vi "PopUpDisplay.vi"(0 "Data":i16[][](array[numeric]), 5 "Plane":i32, 7 "Motion Settings In":T1={"No Motion?"=FALSE, "Motion System"=enum."NI 735x", "Motion Bd ID"=1, "Motion Profile"="SMAC1", "# Axis"=1, "Reverse Z axis?"=TRUE, "SMAC Axis"=0, "scan pair"=enum."y-(x) scan", "RT fps"=6.0, "Steps per mm"=[1000, 1000, 1000, 1000], "Motor Parameters"={"velocity ct/s"=[10000.0, 10000.0, 10000.0, 50000.0], "accel ct/s^2"=[50000.0, 50000.0, 50000.0, 200000.0]}, "One Way Scan"=FALSE, "Reverse One Way Scan"=FALSE, "Global Position (mm)"=[], "Plane"=0, "Distance between\nscan lines (um)"=0.0, "Distance between\nscan planes (um)"=0.0, "number of scan planes"=1, "Total steps in line"=0, "Xtra plane\ndistance  (um)"=100, "Xtra planes "=1, "Add Axis"=FALSE, "overshoot cts"=200, "BKPT Shift"=0, "Scan Start Time (ms)"=0, "ESP VISA"="GPIB::1::INSTR", "3rd Axis"=1, "GL Ref Out"=refnum, "Galil Address"=""} {"3rd Axis" items=["x", "y", "z", "w"]; "Xtra planes" min=1; "Xtra plane\ndistance  (um)" min=0; "Distance between\nscan planes (um)" format="%.2f"; "Distance between\nscan lines (um)" format="%.2f"; "SMAC Axis" items=["None"=0, "Axis 1"=1, "Axis 2"=2, "Axis 3"=3, "Axis 4"=4, "Axis 5"=5, "Axis 6"=6, "Axis 7"=7, "Axis 8"=8, "Vector Space 1"=17, "Vector Space 2"=18, "Vector Space 3"=19, "Vector Space 4"=20]; "Motion Bd ID" min=1 max=32 step=1}, 9 "Digitizer Settings":T5={"Digitizer delay (us) "=0.0, "rf points per line"=2048, "lines per plane"=128, "Samp Rate (Hz)"=100000000.0, "Additional dig delay (us)"=0.0, "Voltage Scale"=0.4, "Pre-Looks"=0, "Offset delay (us)"=0.0, "bits A/D"=8, "Avg Num"=1, "DigTimeOut"=5.0, "Rel Dig Delay"=0.0, "Dig Ch"=0, "LeCroyCluster"={"LeCroy Channels"=[TRUE, FALSE, FALSE, FALSE], "LC read pt offset"=0.0, "Sweep Avg"=FALSE}, "Main Digitizer"=enum."NI Digitizer", "Dig Config"=enum."Single channel", "Digitizer ID Cluster"={"Acqiris/Alazar/SP ID"=[], "NI Instr Handles"=[], "LeCroy VISA"="", "GaGe Handle"={"Handle"=0, "Sample size"=0, "Resolution"=0, "Offset"=0, "Channels"=0, "Boards"=0}, "ATS Ref"="ATS9350", "Acqiris Address"=["PCI::INSTR0"], "ADQRef"=refnum, "adq_cu_ptr"=refnum}, "Trigger Settings"={"Trig Source"=1, "Trig Coupling"=0, "Trig Slope"=0, "Level (mV)"=1500.0}, "Bulk Acq"=FALSE, "Bulk Start Indexes"=[], "Data Ref RF"=refnum, "NI ID/Channel"=[], "Total Dig CH"=1, "Xtra Ann Trig delay (us)"=10.0, "Fix Z Delay?"=FALSE, "One Way Transmission?"=FALSE, "Data Ref Log"=refnum} {"Trigger Settings"."Trig Slope" items=["Positive", "Negative"]; "Trigger Settings"."Level (mV)" format="%.2f"; "Trigger Settings"."Trig Coupling" items=["DC 1 MOhm", "AC 1 MOhm", "DC 50 Ohm", "AC 50 Ohm"]; "Trigger Settings"."Trig Source" items=["Chan 1", "External"]; "Rel Dig Delay" format="%.2f"; "DigTimeOut" format="%.2f"; "Avg Num" min=1; "Offset delay (us)" format="%.2f"; "Additional dig delay (us)" format="%.2f"; "Digitizer delay (us)" format="%.2f"}, 11 "virtual T/R Pairs":i32=1) -> ()   [LabVIEW 2022 SP3]
uses:
  ViewData/-ReadEye/ScaleMethod.ctl
  ViewData/-ReadEye/TypeDefs/TypeofMean.ctl
  Digitizers/-DigitizerRoutines/DigitizerSettings.ctl
  Digitizers/-DigitizerRoutines/Digitizer.ctl
  Digitizers/-DigitizerRoutines/DigConfig.ctl
  Digitizers/-DigitizerRoutines/DigitizerID.ctl
  C:/Windows/System32/ADQAPI_dotNet_helper.dll
  Motion Controllers/NI_controller/-NI_MotionRoutines/MotionParameters.ctl
  Motion Controllers/NI_controller/-NI_MotionRoutines/MotionSys.ctl
  Motion Controllers/-MotionRoutines/ScanAxis.ctl
  Motion Controllers/-MotionRoutines/3rdAxis.ctl
  <vilib>/Utility/miscctls.llb/LVRectTypeDef.ctl
  Motion Controllers/-MotionRoutines/MotionGlobals.vi
panel:
  in  "1-to-1":bool=TRUE
  in  "Flip x?":bool
  in  "Filter Prams":T9={"low cutoff"=5, "order"=81, "high cutoff"=65}
  in  "Type of Mean":T10=enum."No mean"
  in  "Display mode":T11=enum."Log Grey Scale"
  out "Raw data":dbl[][](graph)
  # "Last Completed Plane"
  # "1-D and 2-D B scan settings"
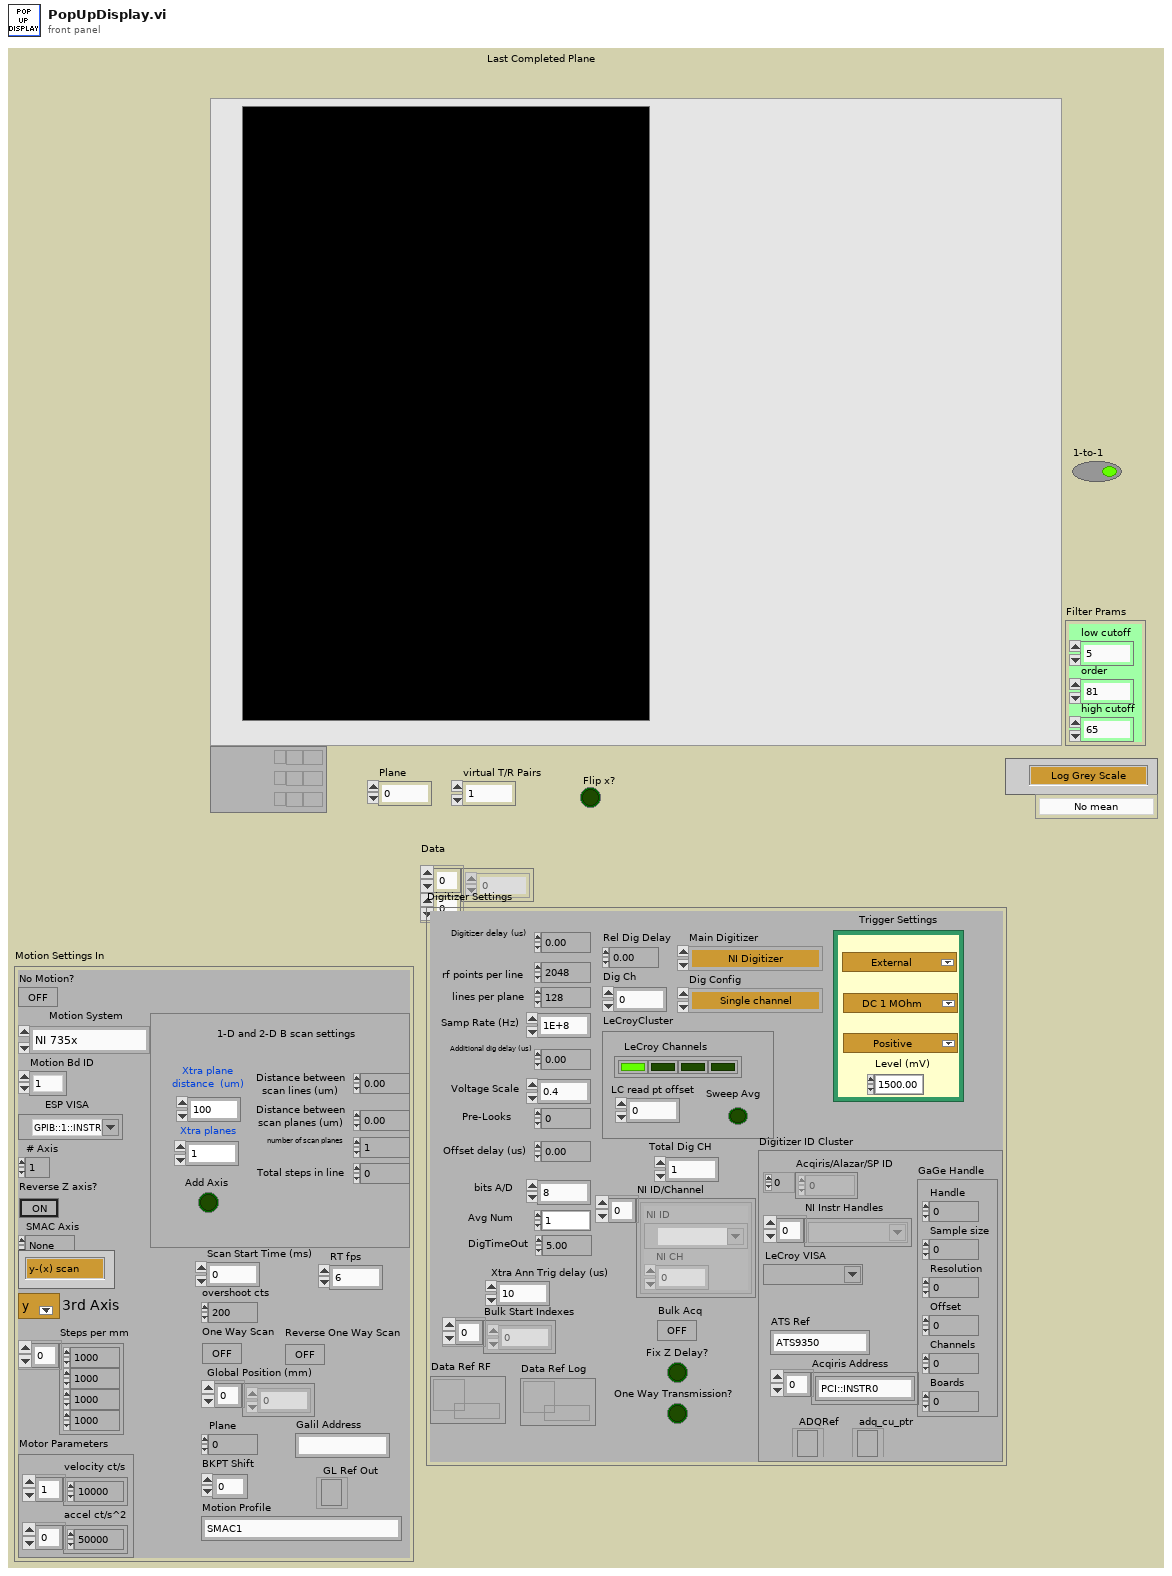
[diagram p1: front panel]
types:
  T1 = typedef "MotionParameters.ctl" = cluster{"No Motion?":bool, "Motion System":T2, "Motion Bd ID":u8, "Motion Profile":string, "# Axis":i8, "Reverse Z axis?":bool, "SMAC Axis":u16, "scan pair":T3, "RT fps":sgl, "Steps per mm":i32[], "Motor Parameters":cluster{"velocity ct/s":dbl[], "accel ct/s^2":dbl[]}, "One Way Scan":bool, "Reverse One Way Scan":bool, "Global Position (mm)":dbl[], "Plane":i32, "Distance between\nscan lines (um)":sgl, "Distance between\nscan planes (um)":sgl, "number of scan planes":i32, "Total steps in line":i32, "Xtra plane\ndistance  (um)":i32, "Xtra planes ":i32, "Add Axis":bool, "overshoot cts":i32, "BKPT Shift":i32, "Scan Start Time (ms)":u32, "ESP VISA":refnum<visa-resource-name>, "3rd Axis":T4, "GL Ref Out":refnum<k7>, "Galil Address":string}
  T2 = typedef "MotionSys.ctl" = enum16{"MM3000", "NI 735x", "Newport ESP", "No Motion Card", "Galil"}
  T3 = typedef "ScanAxis.ctl" = enum16{"y-(x) scan", "x-(y) scan", "z-(x) scan", "z-(y) scan", "y-(z) scan", "x-(z) scan", "w-(x) scan", "w-(y) scan", "w-(z) scan", "x-(w) scan", "y-(w) scan", "z-(w) scan"}
  T4 = typedef "3rdAxis.ctl" = u16
  T5 = typedef "DigitizerSettings.ctl" = cluster{"Digitizer delay (us) ":dbl, "rf points per line":i32, "lines per plane":i32, "Samp Rate (Hz)":dbl, "Additional dig delay (us)":dbl, "Voltage Scale":dbl, "Pre-Looks":i32, "Offset delay (us)":dbl, "bits A/D":i8, "Avg Num":i32, "DigTimeOut":sgl, "Rel Dig Delay":sgl, "Dig Ch":i32, "LeCroyCluster":cluster{"LeCroy Channels":bool[], "LC read pt offset":dbl, "Sweep Avg":bool}, "Main Digitizer":T6, "Dig Config":T7, "Digitizer ID Cluster":T8, "Trigger Settings":cluster{"Trig Source":u16, "Trig Coupling":u16, "Trig Slope":u16, "Level (mV)":dbl}, "Bulk Acq":bool, "Bulk Start Indexes":i32[], "Data Ref RF":refnum<data-value>, "NI ID/Channel":cluster{"NI ID":refnum<k15>, "NI CH":i32}[], "Total Dig CH":i32, "Xtra Ann Trig delay (us)":dbl, "Fix Z Delay?":bool, "One Way Transmission?":bool, "Data Ref Log":refnum<data-value>}
  T6 = typedef "Digitizer.ctl" = enum16{"Acqiris Digitizer", "NI Digitizer", "LeCroy", "GaGe", "AlazarTech", "No Digitizer", "Teledyne"}
  T7 = typedef "DigConfig.ctl" = enum16{"Single channel", "2 Chans w/ 2 Acqiris", "2 Chans w/ 1 Acqiris", "5-CH Pulser New", "5-CH pulser w/ ann array", "5-pass style ann array", "Empty"}
  T8 = typedef "DigitizerID.ctl" = cluster{"Acqiris/Alazar/SP ID":u32[], "NI Instr Handles":refnum<k15>[], "LeCroy VISA":refnum<visa-resource-name>, "GaGe Handle":cluster{"Handle":u32, "Sample size":u32, "Resolution":i32, "Offset":i32, "Channels":u32, "Boards":u32}, "ATS Ref":string, "Acqiris Address":string[], "ADQRef":refnum<k24>, "adq_cu_ptr":refnum<k24>}
  T9 = cluster{"low cutoff":i32, "order":i32, "high cutoff":i32}
  T10 = typedef "TypeofMean.ctl" = enum16{"Mean from lines", "Mean just lines", "Poly Mean", "No mean", "Filter"}
  T11 = typedef "ScaleMethod.ctl" = enum16{"Linear Abs Grey", "Log Grey Scale", "Linear Color Scale", "dB Scale", "Verasonics Doppler"}
  T12 = typedef "LVRectTypeDef.ctl" = cluster{"Left":i16, "Top":i16, "Right":i16, "Bottom":i16}
  T13 = cluster{"Y Scale Offset":dbl, "Y Scale Multi":dbl, "X Scale Offset":dbl, "X Scale Multi":dbl, "Gate Distance":dbl}
  T14 = typedef "LVBoundsTypeDef.ctl" = cluster{"Width":u32, "Height":u32}
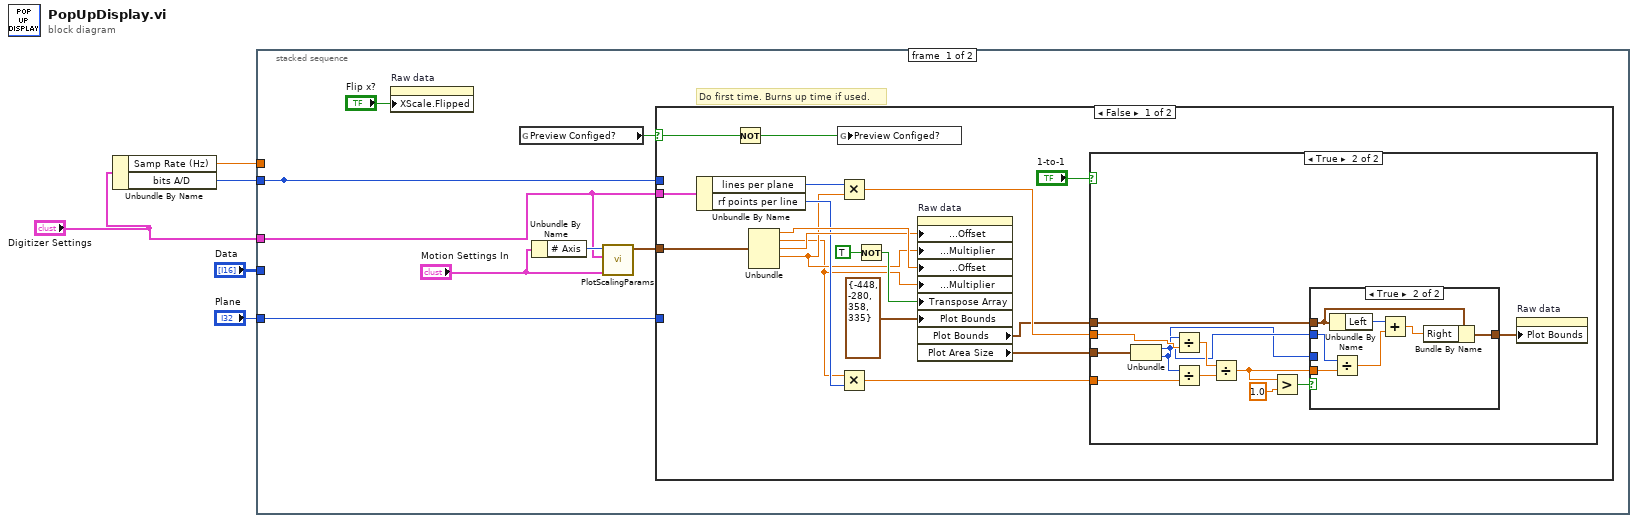
[diagram p0: block diagram]
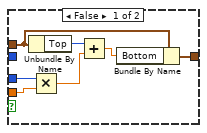
[diagram p3: hidden frame]
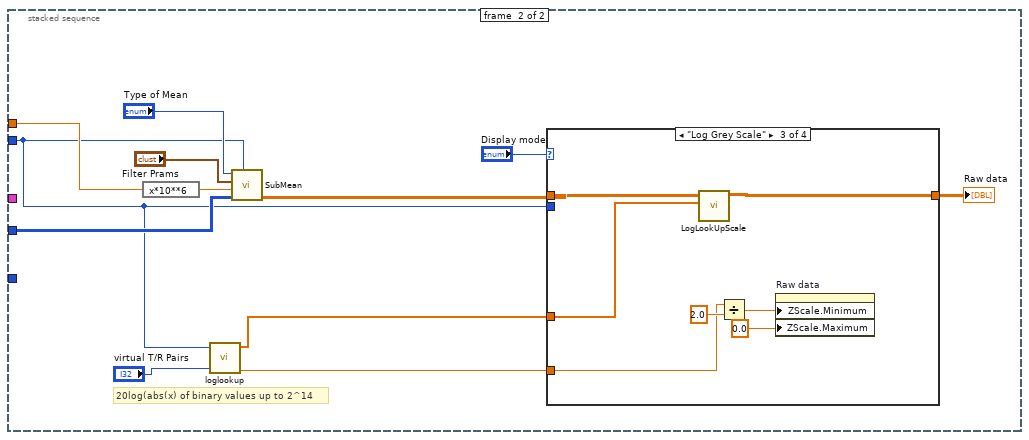
[diagram p5: hidden frame]
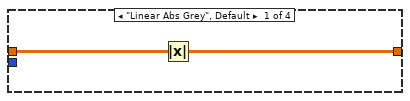
[diagram p6: hidden frame]
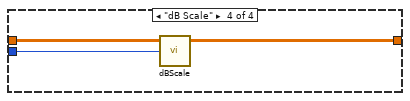
[diagram p8: hidden frame]
diagram:
  n1 = Unbundle By Name("Digitizer Settings") -> ("Samp Rate (Hz)"=w2:dbl, "bits A/D"=w1:i8)
  n2 = stacked-sequence {
    tunnel: "Plane" -> [w13 _]
    tunnel: "Data" -> [_ w67]
    tunnel: "Digitizer Settings" -> [w8 _]
    tunnel: w2 -> [_ w62]
    tunnel: w1 -> [w6 w59]
    tunnel: [w6 _] -> _
    frame #0 {
      # "Do first time. Burns up time if used."
      n3 = property on="Raw data" class="IntGraph (strict)"("XScale.Flipped"="Flip x?") -> ()  [unwired: 2 in, 2 out]
      n4 = global read "MotionGlobals.vi" "Preview Configed?"() -> (w7:bool)
      n5 = Unbundle By Name("Motion Settings In") -> ("# Axis"=w10:i8)
      n6 = call "PlotScalingParams.vi"("Motion Settings In"="Motion Settings In", "Digitizer Settings"=w8, "Scan Axis"=w10) -> ("Cluster"=w12:T13)  [unwired: 6 in, 2 out]
      n7 = case shown="False" w7 {
        selector: w7 -> [w15 _]
        tunnel: w13 -> [_ _]
        tunnel: w12 -> [w31 _]
        tunnel: w8 -> [w30 _]
        tunnel: w6 -> [_ _]
        frame False {
          n8 = Unbundle By Name(w30) -> ("lines per plane"=w22:i32, "rf points per line"=w21:i32)
          n9 = Not(x=w15) -> (.not. x?=w14:bool)
          n10 = Unbundle(w31) -> ("Y Scale Offset"=w29:dbl, "Y Scale Multi"=w19:dbl, "X Scale Offset"=w26:dbl, "X Scale Multi"=w20:dbl)  [unwired: 1 out]
          n11 = global write "MotionGlobals.vi" "Preview Configed?"(w14) -> ()
          n12 = Multiply(x=w22, y=w20) -> (x*y=w25:dbl)
          n13 = Multiply(x=w19, y=w21) -> (x*y=w24:dbl)
          n14 = Not(x=TRUE ("view")) -> (.not. x?=w27:bool)
          n15 = property on="Raw data" class="IntGraph (strict)"("X Scale.Offset and Multiplier:Offset"=w26, "X Scale.Offset and Multiplier:Multiplier"=w20, "Y Scale.Offset and Multiplier:Offset"=w29, "Y Scale.Offset and Multiplier:Multiplier"=w19, "Transpose Array"=w27, "Plot Bounds"=T12 {"Left"=-448, "Top"=-280, "Right"=358, "Bottom"=335} ("Plot Area Bounds")) -> ("Plot Bounds"=w18:T12, "Plot Area Size"=w23:T14)  [unwired: 2 in, 2 out]
          n16 = case shown="True" "1-to-1" {
            tunnel: w25 -> [_ w43]
            tunnel: w24 -> [_ w42]
            tunnel: w23 -> [_ w33]
            tunnel: w18 -> [_ w32]
            frame False {
            }
            frame True {
              n17 = Unbundle(w33) -> ("Width"=w37:u32, "Height"=w35:u32)
              n18 = Divide(x=w37, y=w43) -> (x/y=w41:dbl)
              n19 = Divide(x=w35, y=w42) -> (x/y=w40:dbl)
              n20 = Divide(x=w41, y=w40) -> (x/y=w36:dbl)
              n21 = Greater?(x=w36, y=1.0) -> (0:w39:bool)
              n22 = case shown="True" w39 {
                tunnel: w37 -> [_ w57]
                tunnel: w36 -> [w50 w56]
                tunnel: w35 -> [w49 _]
                tunnel: w32 -> [w44 w55]
                tunnel: [w45 w51] -> w34
                frame False {
                  n23 = Unbundle By Name(w44) -> ("Top"=w48:i16)
                  n24 = Multiply(x=w49, y=w50) -> (x*y=w46:dbl)
                  n25 = Add(x=w48, y=w46) -> (x+y=w47:dbl)
                  n26 = Bundle By Name(cluster=w44, "Bottom"=w47) -> (w45:T12)
                }
                frame True {
                  n27 = Unbundle By Name(w55) -> ("Left"=w53:i16)
                  n28 = Divide(x=w57, y=w56) -> (x/y=w54:dbl)
                  n29 = Add(x=w53, y=w54) -> (x+y=w52:dbl)
                  n30 = Bundle By Name(cluster=w55, "Right"=w52) -> (w51:T12)
                }
              }
              n31 = property on="Raw data" class="IntGraph (strict)"("Plot Bounds"=w34) -> ()  [unwired: 2 in, 2 out]
            }
          }
        }
        frame True {
        }
      }
    }
    frame #1 {
      # "20log(abs(x) of binary values up to 2^14"
      n32 = expression code="x*10**6"(w62) -> (w63:dbl)
      n33 = call "loglookup.vi"("A/D bits"=w59, "virtual T/R Pairs"="virtual T/R Pairs") -> ("Log Lookup"=w60:sgl[], "Minimum dB"=w58:dbl)  [unwired: 1 in, 2 out]
      n34 = call "SubMean.vi"("Bit Depth"=w59, "Scan Data In"=w67, "Samp Rate (MHz)"=w63, "Filter Prams"="Filter Prams", "Type of Mean"="Type of Mean") -> ("Array"=w69:dbl[][])  [unwired: 1 in, 2 out]
      n35 = case shown="\"Log Grey Scale\"" "Display mode" {
        tunnel: [w70 w72 w78 w81] -> w68
        tunnel: w69 -> [w71 w72 w79 w82]
        tunnel: w59 -> [_ _ _ w80]
        tunnel: w60 -> [_ _ w74 _]
        tunnel: w58 -> [_ _ w73 _]
        frame "Linear Abs Grey", Default {
          n36 = Absolute Value(x=w71) -> (abs(x)=w70:dbl[][])
        }
        frame "Linear Color Scale" {
        }
        frame "Log Grey Scale" {
          n37 = call "LogLookUpScale.vi"("Log Lookup"=w74, "Array in"=w79) -> ("Array out"=w78:sgl[][])  [unwired: 9 in]
          n38 = Divide(x=w73, y=sgl 2.0) -> (x/y=w77:dbl)
          n39 = property on="Raw data" class="IntGraph (strict)"("ZScale.Minimum"=w77, "ZScale.Maximum"=0.0 ("Z Scale.Range:Maximum")) -> ()  [unwired: 2 in, 2 out]
        }
        frame "dB Scale" {
          n40 = call "dBScale.vi"("Bit Depth"=w80, "Data In"=w82) -> ("Data Out"=w81:dbl[][])  [unwired: 3 in]
        }
      }
      "Raw data" <- w68
    }
  }
